vi "1_Connect_and_read_serial_number.vi"() -> ()   [LabVIEW 2014]
uses:
  <vilib>/Swabian Instruments/Pulse Streamer/PulseStreamer/helpers/typedef_DeviceInfo.ctl
  <vilib>/Swabian Instruments/Pulse Streamer/PulseStreamer/PulseStreamer/PulseStreamer.lvclass
  <vilib>/Swabian Instruments/Pulse Streamer/PulseStreamer/PulseStreamer.lvlib
panel:
  out "IP address":string
  out "Descriptions":T1[](array[typedef])
  in  "search_serial":string
  out "FPGA ID":string
  out "SerialNumber":string
  out "FirmwareVersion":string
  out "error out":errorcluster
  # "This very simple example shows how to establish connection to Pulse Streamer.\nWhat it does:\n - Searches the Pulse Streamers on the network\n - Connects to the first found Pulse Streamer by the IP address.\n - Reads firmware version and serial number (network MAC address)."
  # "NETWORK SCAN RESULTS    \n   -   requires firmware version 1.2 or higher\n\nYou can search for a Pulse Streamer with a specific serial number by entering it in the \"search_serial\" field.\nWhen this field is empty, all discovered devices are listed."
  # "Connecting to a first discovered PulseStreamer"
  # "Default host name is 'pulsestreamer' when\nusing DHCP (please connect the LAN cable\nbefore powering on the device).\nOtherwise the fallback IP is 169.254.8.2 if\nthe device is connected directly to the computer."
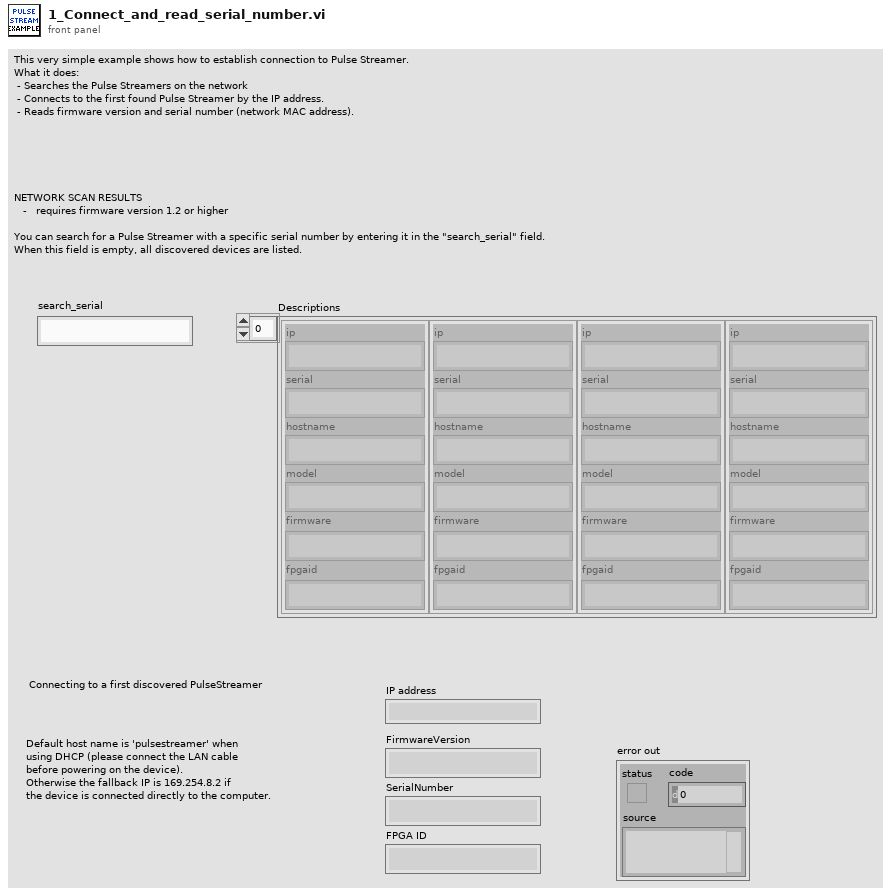
[diagram p1: front panel]
types:
  T1 = typedef "PulseStreamer.lvlib/typedef_DeviceInfo.ctl" = cluster{"ip":string, "serial":string, "hostname":string, "model":string, "firmware":string, "fpgaid":string}
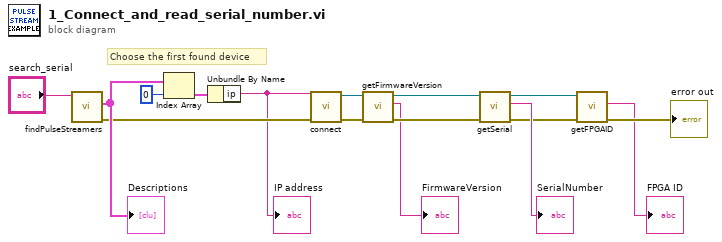
[diagram p0: block diagram]
diagram:
  # "Choose the first found device"
  n1 = call <vilib>:"findPulseStreamers.vi"("search_serial"="search_serial") -> ("error out"=w4:errorcluster, "Descriptions"=w5:T1[])  [unwired: 9 in]
  "Descriptions" <- w5
  n2 = Index Array(array=w5, index=0) -> (element=w2:T1)
  n3 = Unbundle By Name(w2) -> ("ip"=w1:string)
  "IP address" <- w1
  n4 = call <vilib>:"connect.vi"("error in (no error)"=w4, "ip"=w1) -> ("error out"=w16:errorcluster, "Pulse Streamer out"=w15:refnum<class "PulseStreamer.lvclass">)  [unwired: 8 in]
  n5 = call <vilib>:"getFirmwareVersion.vi"("error in (no error)"=w16, "Pulse Streamer in"=w15) -> ("error out"=w14:errorcluster, "Version"=→"FirmwareVersion":string, "Pulse Streamer out"=w13:refnum<class "PulseStreamer.lvclass">)  [unwired: 7 in]
  n6 = call <vilib>:"getSerial.vi"("error in (no error)"=w14, "Pulse Streamer in"=w13) -> ("error out"=w10:errorcluster, "Serial"=→"SerialNumber":string, "Pulse Streamer out"=w8:refnum<class "PulseStreamer.lvclass">)  [unwired: 7 in]
  n7 = call <vilib>:"getFPGAID.vi"("error in (no error)"=w10, "Pulse Streamer in"=w8) -> ("error out"=→"error out":errorcluster, "FPGA ID"=→"FPGA ID":string)  [unwired: 7 in, 1 out]
